vi "check_error.vi"(8 "error in":errorcluster) -> (0 "error out":errorcluster)   [LabVIEW 2010]
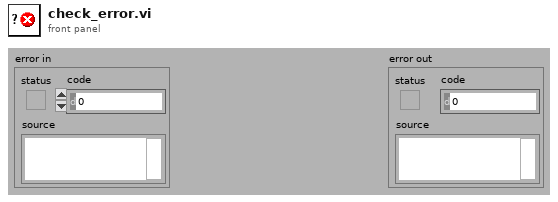
[diagram p1: front panel]
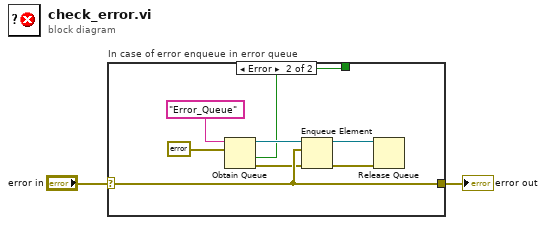
[diagram p0: block diagram]
diagram:
  n1 = case "In case of error enqueue in error queue" shown="Error" "error in" {
    selector: "error in" -> [w3 w8]
    tunnel: [w3 w8] -> w1
    tunnel: [_ w4] -> _
    frame No Error {
    }
    frame Error {
      n2 = Obtain Queue(name (unnamed)="Error_Queue", element data type=errorcluster {"status"=FALSE, "code"=0, "source"=""} ("error in (no error)")) -> (queue out=w9:refnum<queue>, created new?=w4:bool, error out=w5:errorcluster)  [unwired: 3 in]
      n3 = Enqueue Element(queue=w9, element=w8, error in (no error)=w5) -> (queue out=w7:refnum<queue>, error out=w6:errorcluster)  [unwired: 1 in, 1 out]
      n4 = Release Queue(queue=w7, error in (no error)=w6) -> ()  [unwired: 1 in, 3 out]
    }
  }
  "error out" <- w1
